vi "ROBO_Pendubot.vi"() -> ()   [LabVIEW 2012]
uses:
  <vilib>/addons/Control Design/_Model Conversions/NI_CD_Continuous and Discrete.lvlib
  <vilib>/addons/Control Design/_Model Conversions/Continuous and Discrete.llb/Continuous and Discrete SubVI/cd_Convert Continuous to Discrete (SS).vi
  <vilib>/addons/Control Design/_Model Construction/NI_LinSys_Model Creation.lvlib
  <vilib>/addons/Control Design/_Model Construction/Model Creation.llb/Model Creation SubVI/cd_Create State Space Model.vi
  <vilib>/addons/Control Design/_State Feedback Control/NI_CD_State Feedback Control.lvlib
  <vilib>/addons/Control Design/_Dynamic Analysis/NI_CD_Dynamic Analysis.lvlib
  <vilib>/addons/Control Design/_Dynamic Analysis/Dynamic Analysis.llb/Dynamic Analysis subVI/cd_Poles (State-Space).vi
  <vilib>/addons/Control Design/_Utility/NI_CD_Model Viewer.lvlib
  <vilib>/addons/Control Design/_Utility/Model Viewer.llb/Model Viewer SubVI/cd_Draw State-Space Equation (SS).vi
panel:
  out "Discrete Model Out":picture
  out "System Poles":cdb[](array[numeric])=[1.2142841528821395+0.0i, 0.8147971273698099+0.0i, 0.9518587677710494+0.0i, 1.0+0.0i] format="%#.2g"
  out "Optimal Gain":dbl[](array[numeric])=[-0.14906178101626644, 0.17686358569380023, 1.1761652926773682, -0.039275718443801] format="%.2f"
  in  "Desired Poles":cdb[](array[numeric])=[-5.0+0.0i, -5.0+0.0i, -20.0+0.0i, -15.0+0.0i] format="%#.2g"
  in  "Discrete Mode":bool=TRUE
  in  "Sampling Time (s)":dbl=0.1
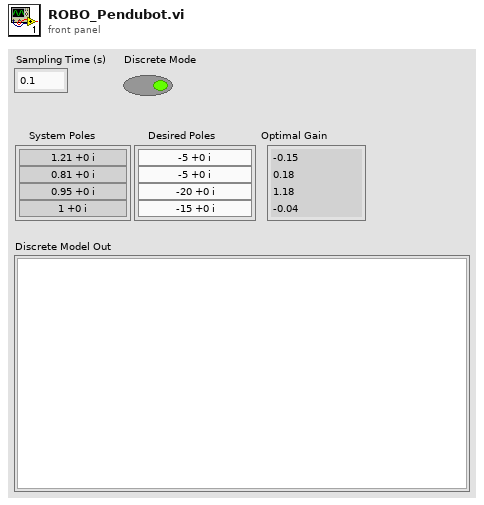
[diagram p1: front panel]
types:
  T1 = typedef "NI_LinSys_Model Typedefs.lvlib/CD State Space Model (MIMO).ctl" = cluster{"properties":T2, "A":dbl[][], "B":dbl[][], "C":dbl[][], "D":dbl[][], "StateNames":string[], "Transport Delay":dbl[][]}
  T2 = typedef "NI_LinSys_Model Typedefs.lvlib/CD General Elements.ctl" = cluster{"Model name":string, "Input names":string[], "Output names":string[], "Input Delays":dbl[], "Output Delays":dbl[], "Sampling Time":dbl, "Notes":string}
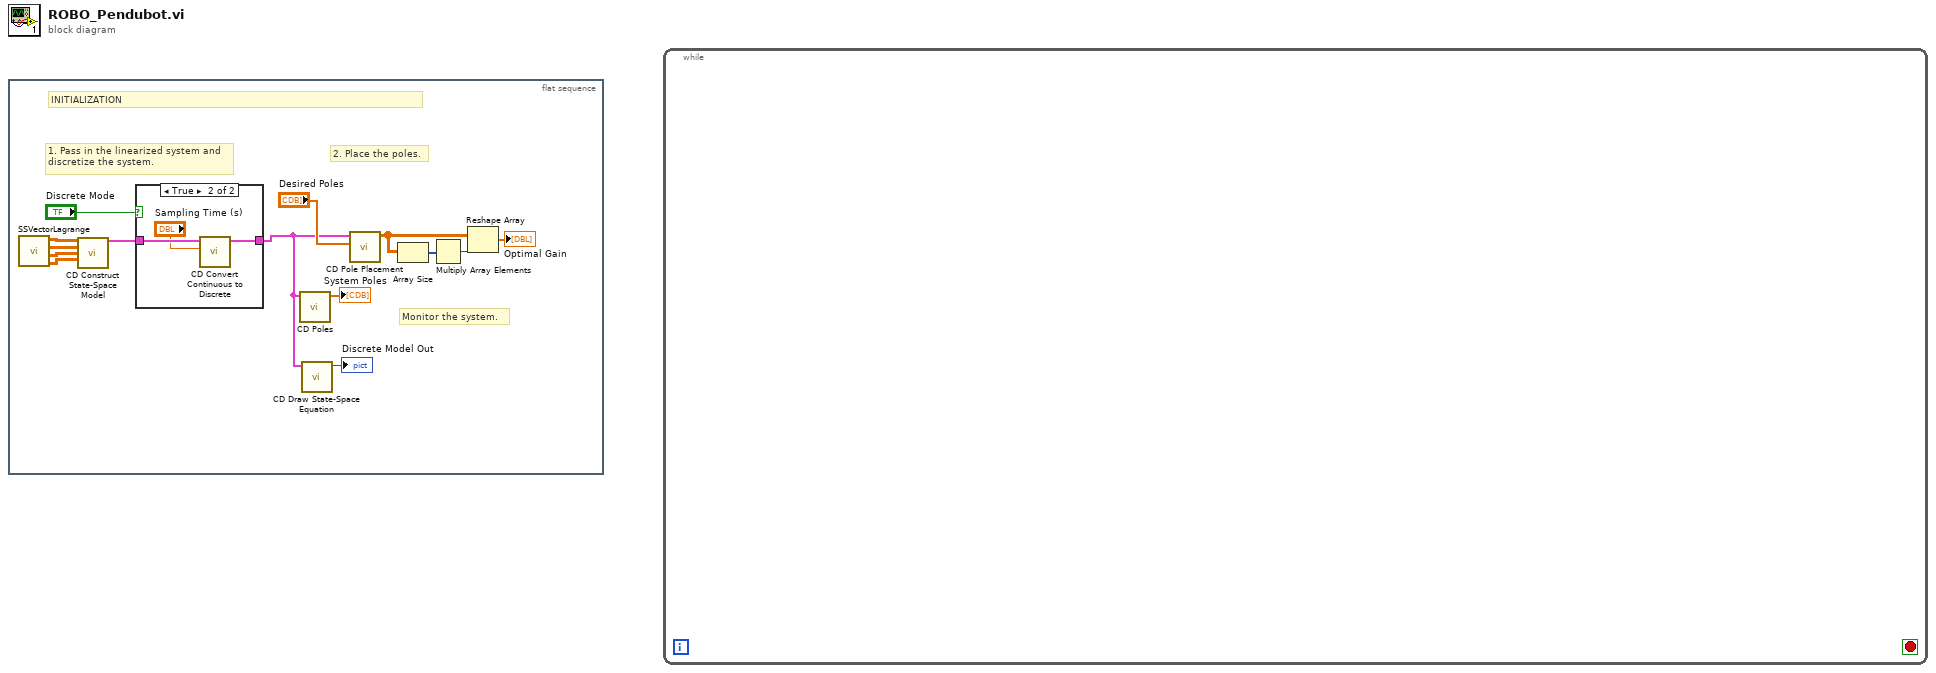
[diagram p0: block diagram]
diagram:
  n1 = flat-sequence {
    frame #0 {
      # "Monitor the system."
      # "2. Place the poles."
      # "1. Pass in the linearized system and\ndiscretize the system."
      # "INITIALIZATION"
      n2 = call "SSVectorLagrange.vi"() -> ("D"=w9:dbl[][], "C"=w10:dbl[][], "B"=w11:dbl[][], "A"=w12:dbl[][])  [unwired: 5 in]
      n3 = call-poly <vilib>:"CD Construct State-Space Model.vi"("A"=w12, "B"=w11, "C"=w10, "D"=w9) -> ("State-Space Model"=w14:T1)  [unwired: 10 in, 1 out]
      n4 = case shown="True" "Discrete Mode" {
        tunnel: w14 -> [w15 w18]
        tunnel: [w15 w16] -> w1
        frame False {
        }
        frame True {
          n5 = call-poly <vilib>:"CD Convert Continuous to Discrete.vi"("Sampling Time (s)"="Sampling Time (s)", "Continuous State-Space Model"=w18) -> ("Discrete State-Space Model"=w16:T1)  [unwired: 7 in, 2 out]
        }
      }
      n6 = call-poly <vilib>:"CD Poles.vi"("State-Space Model"=w1) -> ("Poles"=→"System Poles":cdb[])  [unwired: 9 in, 1 out]
      n7 = call-poly <vilib>:"CD Draw State-Space Equation.vi"("State-Space Model"=w1) -> ("Equation"=→"Discrete Model Out":picture)  [unwired: 8 in, 2 out]
      n8 = call <vilib>:"CD Pole Placement.vi"("Poles"="Desired Poles", "State-Space Model"=w1) -> ("Gain"=w4:dbl[][])  [unwired: 7 in, 2 out]
      n9 = Array Size(array=w4) -> (size(s)=w7:i32[])
      n10 = Multiply Array Elements(1:w7) -> (0:w6:i32)
      n11 = Reshape Array(w4, w6) -> (→"Optimal Gain":dbl[])
    }
  }
  n12 = while {
    stop <- _ stop-if-true
  }
